vi "Write Port.vi"(0 "Cypress in":refnum<class "Cypress.lvclass">, 5 "VISA resource name":refnum<visa-resource-name>, 9 "Port":u16, 11 "error in (no error)":errorcluster, 12 "Set Port":bool[](array[boolean])) -> (4 "Cypress out":refnum<class "Cypress.lvclass">, 6 "VISA resource name out":refnum<visa-resource-name>, 15 "error out":errorcluster)   [LabVIEW 2020, in "Cypress.lvclass"]
uses:
  Cypress.lvclass
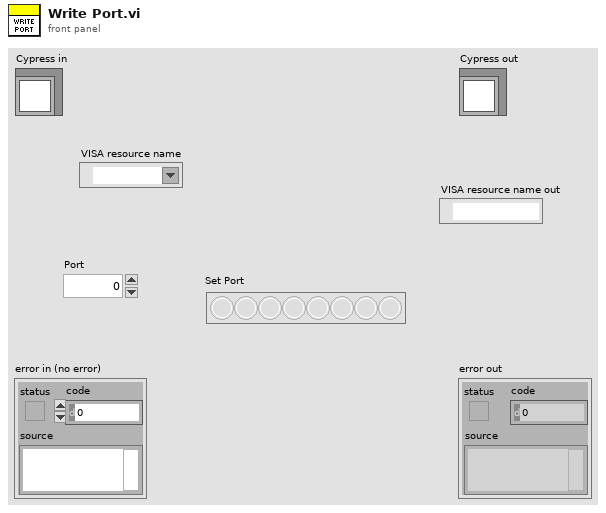
[diagram p1: front panel]
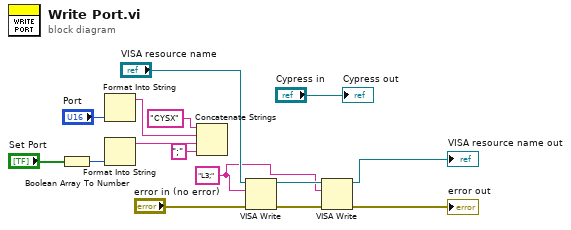
[diagram p0: block diagram]
diagram:
  w4 = "L3;" ("write buffer")
  n1 = Boolean Array To Number(Boolean array="Set Port") -> (number=w11:u32)
  n2 = Format Into String("Port") -> (resulting string=w8:string)  [unwired: 3 in, 1 out]
  n3 = Format Into String(w11) -> (resulting string=w7:string)  [unwired: 3 in, 1 out]
  n4 = Concatenate Strings("CYSX" ("string"), w8, w7, ";" ("string")) -> ()  [unwired: 1 out]
  n5 = VISA Write(VISA resource name="VISA resource name", write buffer=w4, error in (no error)="error in (no error)") -> (VISA resource name out=w5:refnum<visa-resource-name>, error out=w3:errorcluster)  [unwired: 1 out]
  n6 = VISA Write(VISA resource name=w5, write buffer=w4, error in (no error)=w3) -> (VISA resource name out=→"VISA resource name out":refnum<visa-resource-name>, error out=→"error out":errorcluster)  [unwired: 1 out]
  "Cypress out" <- "Cypress in"
